vi "Chirp_substitution.vi"() -> ()   [LabVIEW 2009]
uses:
  <vilib>/Analysis/2dsp.llb/Real FFT.vi
  <vilib>/Utility/file.llb/Read From Spreadsheet File (DBL).vi
  <vilib>/Analysis/NI_AALPro.lvlib
panel:
  in  "Start point":i32=8000
  in  "Points replace":i32=6000
  out "oscilloscope data":dbl[](array[numeric])
  out "deleted portion":dbl[](array[numeric])
  in  "Chirp start (MHz)":ext=2.5
  in  "Filter up to (MHz)":ext=2.5
  in  "ns/div":u32
  in  "ps/point":u32
  out "Final array":ext[][](array[numeric])
  out "Data":dbl[](array[numeric])
  out "XY Graph 5":cluster{ext[], dbl[]}(graph)
  out "FFT (Im)":dbl[](array[numeric])
  out "FFT (Re)":dbl[](array[numeric])
  out "size(s)":i32
  out "Oscilloscope graph":dbl[](graph)
  # "(~6000 points)"
  # "(~8000 points)"
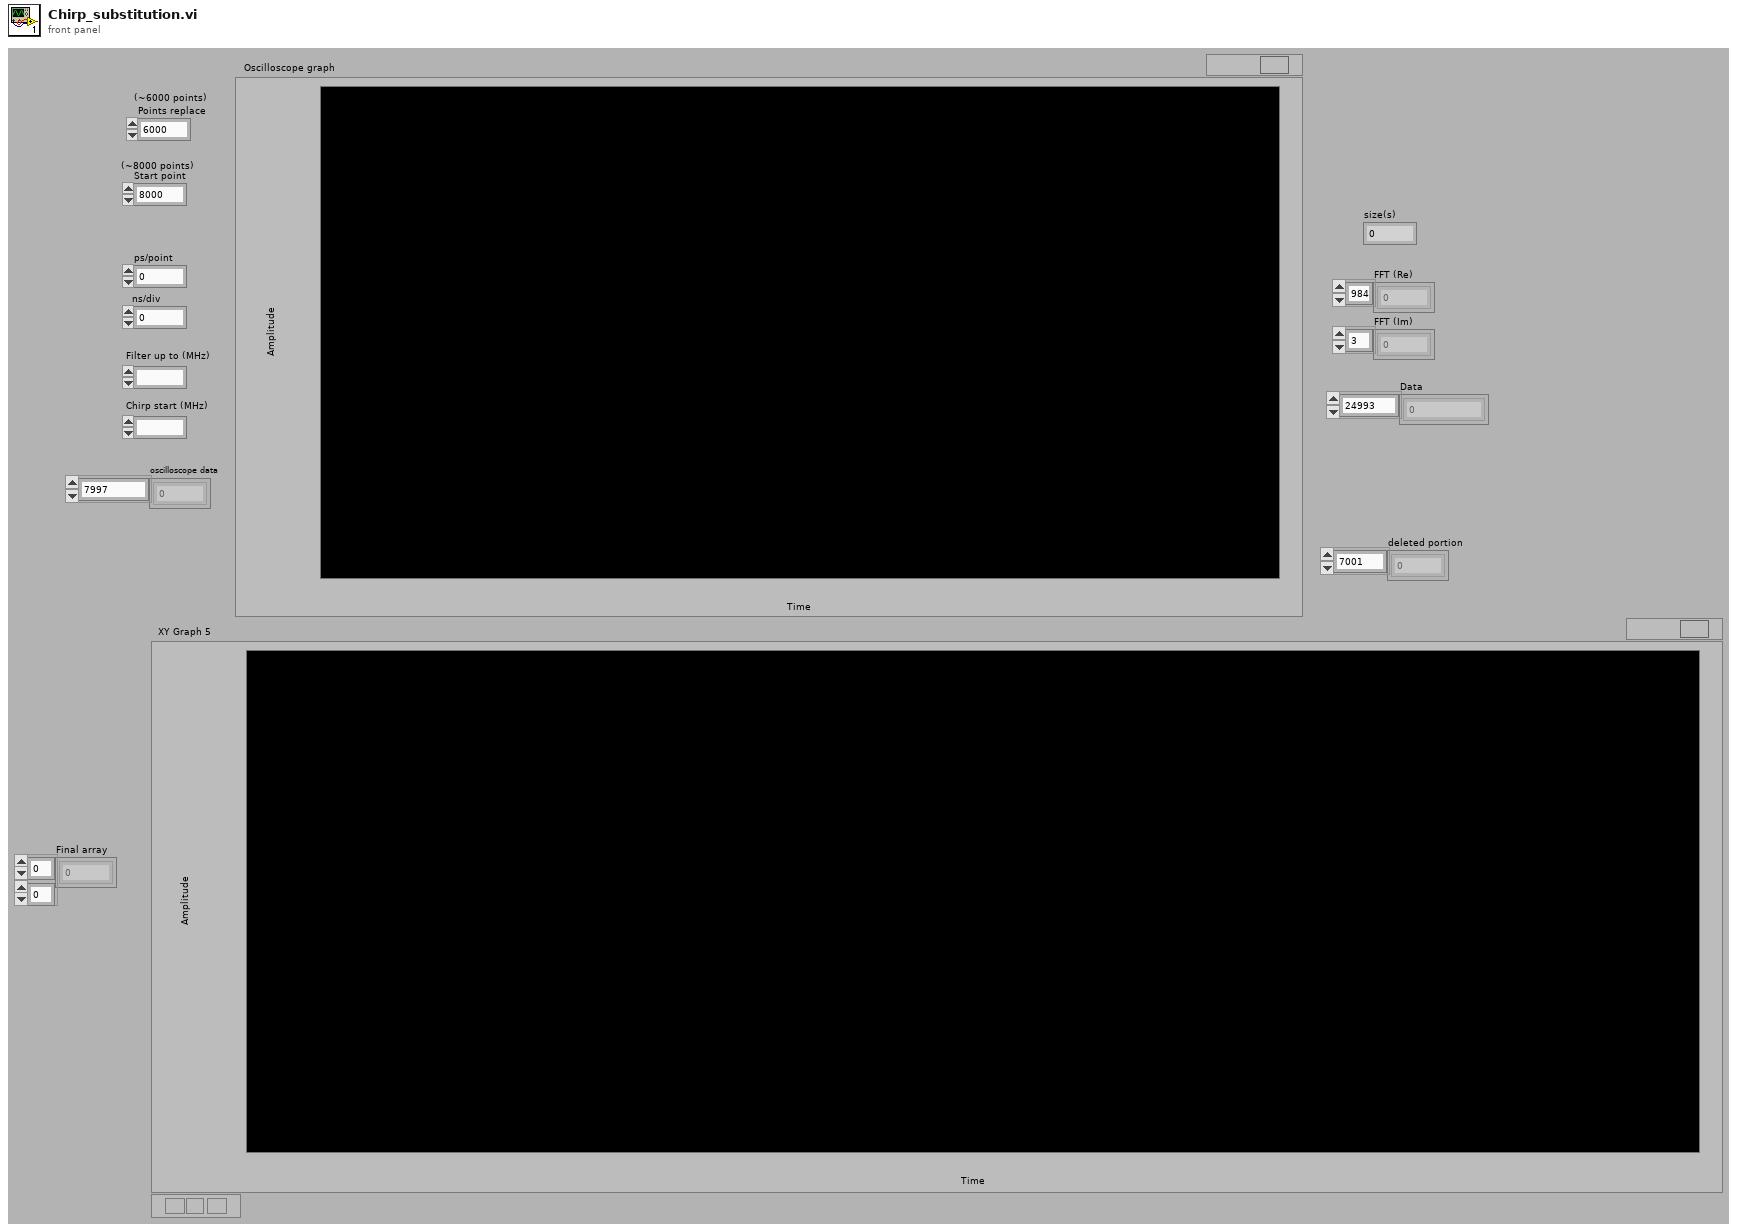
[diagram p1: front panel]
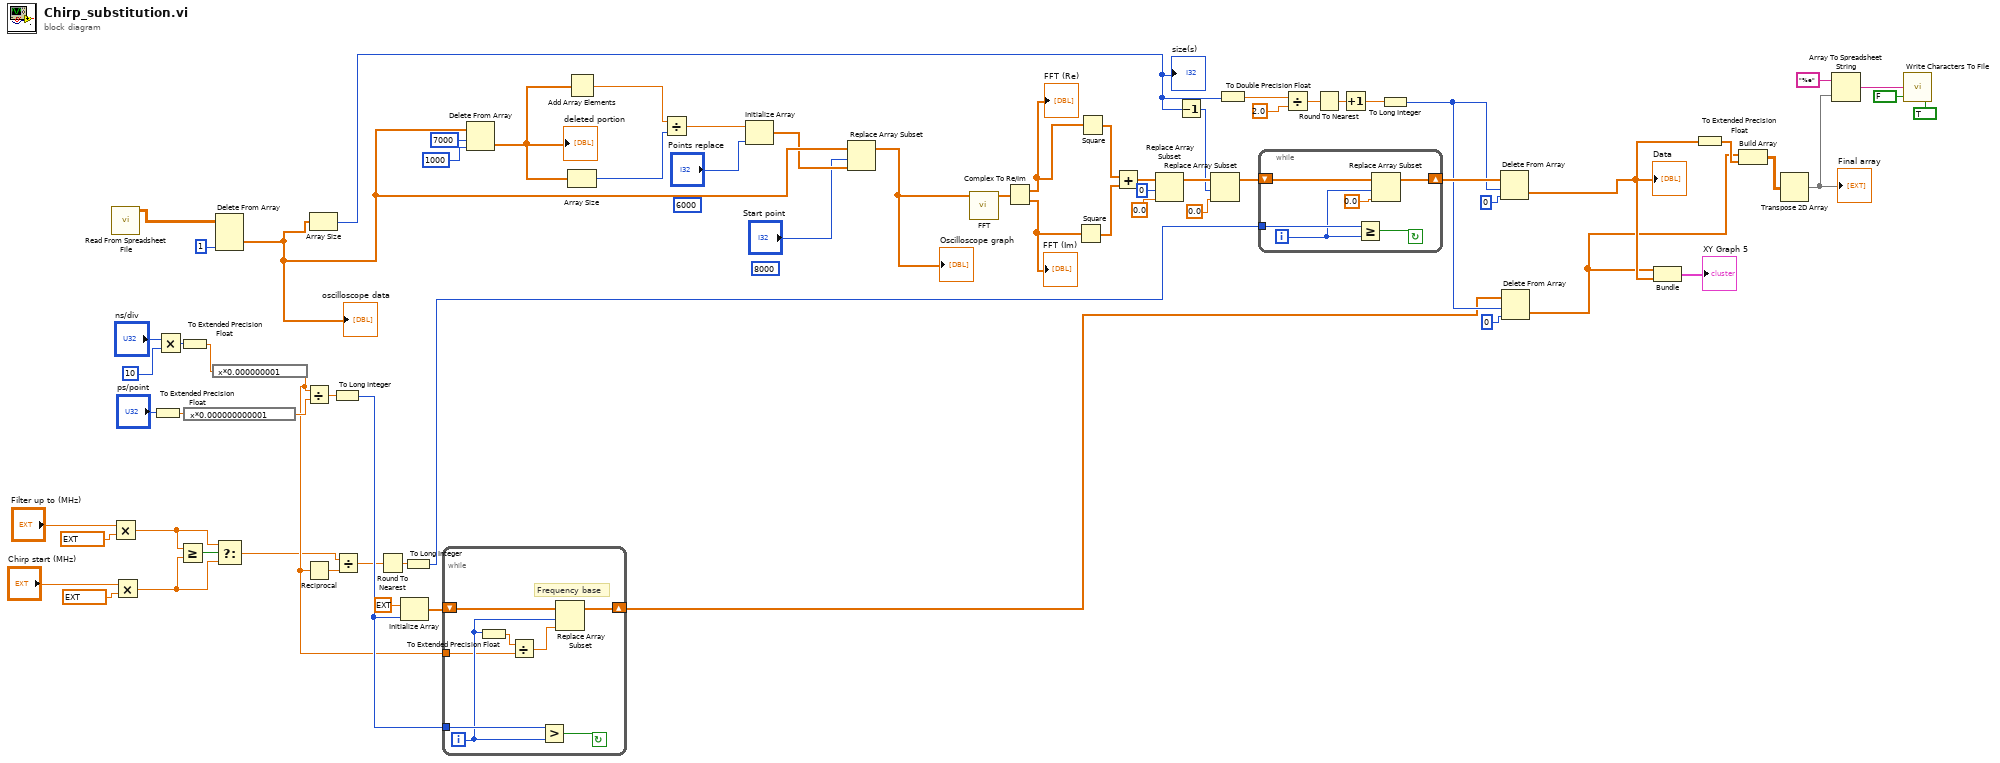
[diagram p0: block diagram]
diagram:
  (unwired) 8000 ("index")
  (unwired) 6000 ("dimension size")
  n1 = call-poly <vilib>:"Read From Spreadsheet File.vi"() -> ("all rows"=w15:dbl[][])  [unwired: 7 in, 4 out]
  n2 = Multiply(x="Filter up to (MHz)", y=ext 1000000.0) -> (x*y=w20:ext)
  n3 = Multiply(x="Chirp start (MHz)", y=ext 1000000.0) -> (x*y=w17:ext)
  n4 = To Extended Precision Float(1:"ps/point") -> (0:w29:ext)
  n5 = Multiply(x="ns/div", y=u32 10) -> (x*y=w38:u32)
  n6 = Greater Or Equal?(x=w20, y=w17) -> (x >= y?=w28:bool)
  n7 = To Extended Precision Float(1:w38) -> (0:w30:ext)
  n8 = expression code="x*0.000000000001"(w29) -> (w31:ext)
  n9 = expression code="x*0.000000001"(w30) -> (w27:ext)
  n10 = Delete From Array(array=w15, index (col)=1 ("disabled index (col)")) -> (deleted portion=w5:dbl[])  [unwired: 2 in, 1 out]
  "oscilloscope data" <- w5
  n11 = Select(t=w20, s=w28, f=w17) -> (s? t:f=w25:ext)
  n12 = Divide(x=w27, y=w31) -> (x/y=w37:ext)
  n13 = Reciprocal(x=w27) -> (1/x=w26:ext)
  n14 = Array Size(array=w5) -> (size(s)=w13:i32)
  "size(s)" <- w13
  n15 = To Long Integer(number=w37) -> (32bit integer=w32:i32)
  n16 = Divide(x=w25, y=w26) -> (x/y=w24:ext)
  n17 = Round To Nearest(number=w24) -> (nearest integer value=w23:ext)
  n18 = Initialize Array(ext 0.0 ("element"), w32) -> (w33:ext[])
  n19 = To Long Integer(number=w23) -> (32bit integer=w16:i32)
  n20 = while {
    tunnel: w32 -> [w77]
    shift-right: [w75] -> w12
    shift-left: w33 -> [w76]
    tunnel: w27 -> [w72]
    i -> [w74]
    stop <- w78 continue-if-true
    # "Frequency base"
    n21 = To Extended Precision Float(1:w74) -> (0:w73:ext)
    n22 = Divide(x=w73, y=w72) -> (x/y=w71:ext)
    n23 = Greater?(x=w77, y=w74) -> (0:w78:bool)
    n24 = Replace Array Subset(array=w76, new element=w71, index=w74) -> (w75:ext[])
  }
  n25 = Delete From Array(array=w5, length=7000, index=1000) -> (deleted portion=w9:dbl[])  [unwired: 1 out]
  "deleted portion" <- w9
  n26 = Add Array Elements(numeric array=w9) -> (sum=w8:dbl)
  n27 = Array Size(array=w9) -> (size(s)=w7:i32)
  n28 = Divide(x=w8, y=w7) -> (x/y=w6:dbl)
  n29 = Initialize Array(w6, "Points replace") -> (w4:dbl[])
  n30 = Replace Array Subset(array=w5, new element=w4, index="Start point") -> (w3:dbl[])
  "Oscilloscope graph" <- w3
  n31 = call-poly <vilib>:"FFT.vi"("X"=w3) -> ("FFT {X}"=w70:cdb[])  [unwired: 9 in, 1 out]
  n32 = Complex To Re/Im(x + iy=w70) -> (x=w69:dbl[], y=w68:dbl[])
  "FFT (Re)" <- w69
  "FFT (Im)" <- w68
  n33 = Square(x=w68) -> (x^2=w66:dbl[])
  n34 = Square(x=w69) -> (x^2=w67:dbl[])
  n35 = Add(x=w67, y=w66) -> (x+y=w57:dbl[])
  n36 = Replace Array Subset(array=w57, new element=0.0 ("new element/subarray"), index=0) -> (w56:dbl[])
  n37 = Decrement(x=w13) -> (x-1=w55:i32)
  n38 = Replace Array Subset(array=w56, new element=0.0 ("new element/subarray"), index=w55) -> (w52:dbl[])
  n39 = To Double Precision Float(number=w13) -> (double precision float=w50:dbl)
  n40 = while {
    tunnel: w16 -> [w83]
    shift-right: [w81] -> w51
    shift-left: w52 -> [w82]
    i -> [w80]
    stop <- w84 continue-if-true
    n41 = Greater Or Equal?(x=w83, y=w80) -> (x >= y?=w84:bool)
    n42 = Replace Array Subset(array=w82, new element=0.0 ("new element/subarray"), index=w80) -> (w81:dbl[])
  }
  n43 = Divide(x=w50, y=2.0) -> (x/y=w48:dbl)
  n44 = Round To Nearest(number=w48) -> (nearest integer value=w47:dbl)
  n45 = Increment(x=w47) -> (x+1=w46:dbl)
  n46 = To Long Integer(number=w46) -> (32bit integer=w41:i32)
  n47 = Delete From Array(array=w51, length=w41, index=0) -> (deleted portion=w44:dbl[])  [unwired: 1 out]
  "Data" <- w44
  n48 = Delete From Array(array=w12, length=w41, index=0) -> (deleted portion=w40:ext[])  [unwired: 1 out]
  n49 = Bundle(w40, w44) -> (→"XY Graph 5":cluster{ext[], dbl[]})  [unwired: 1 in]
  n50 = To Extended Precision Float(1:w44) -> (0:w43:ext[])
  n51 = Build Array(w40, w43) -> (w53:ext[][])
  n52 = Transpose 2D Array(2D array=w53) -> (transposed array=w63:ext[][])
  "Final array" <- w63
  n53 = Array To Spreadsheet String(array=w63, 3:"%e") -> (spreadsheet string=w60:string)  [unwired: 1 in]
  n54 = call <vilib>:"Write Characters To File.vi"("convert eol? (no:F)"=TRUE, "append to file? (new file:F)"=FALSE, "character string"=w60) -> ()  [unwired: 2 in, 1 out]
